vi "Data Save.vi"(11 "Data In":T2) -> (2 "Number":i32, 3 "Data Out":T2)   [LabVIEW 2020]
uses:
  Alin/QMH/000 Module Data Type.ctl
  Alin/QMH/Queue Message.ctl
  <vilib>/Utility/miscctls.llb/LVMapReplaceAction.ctl
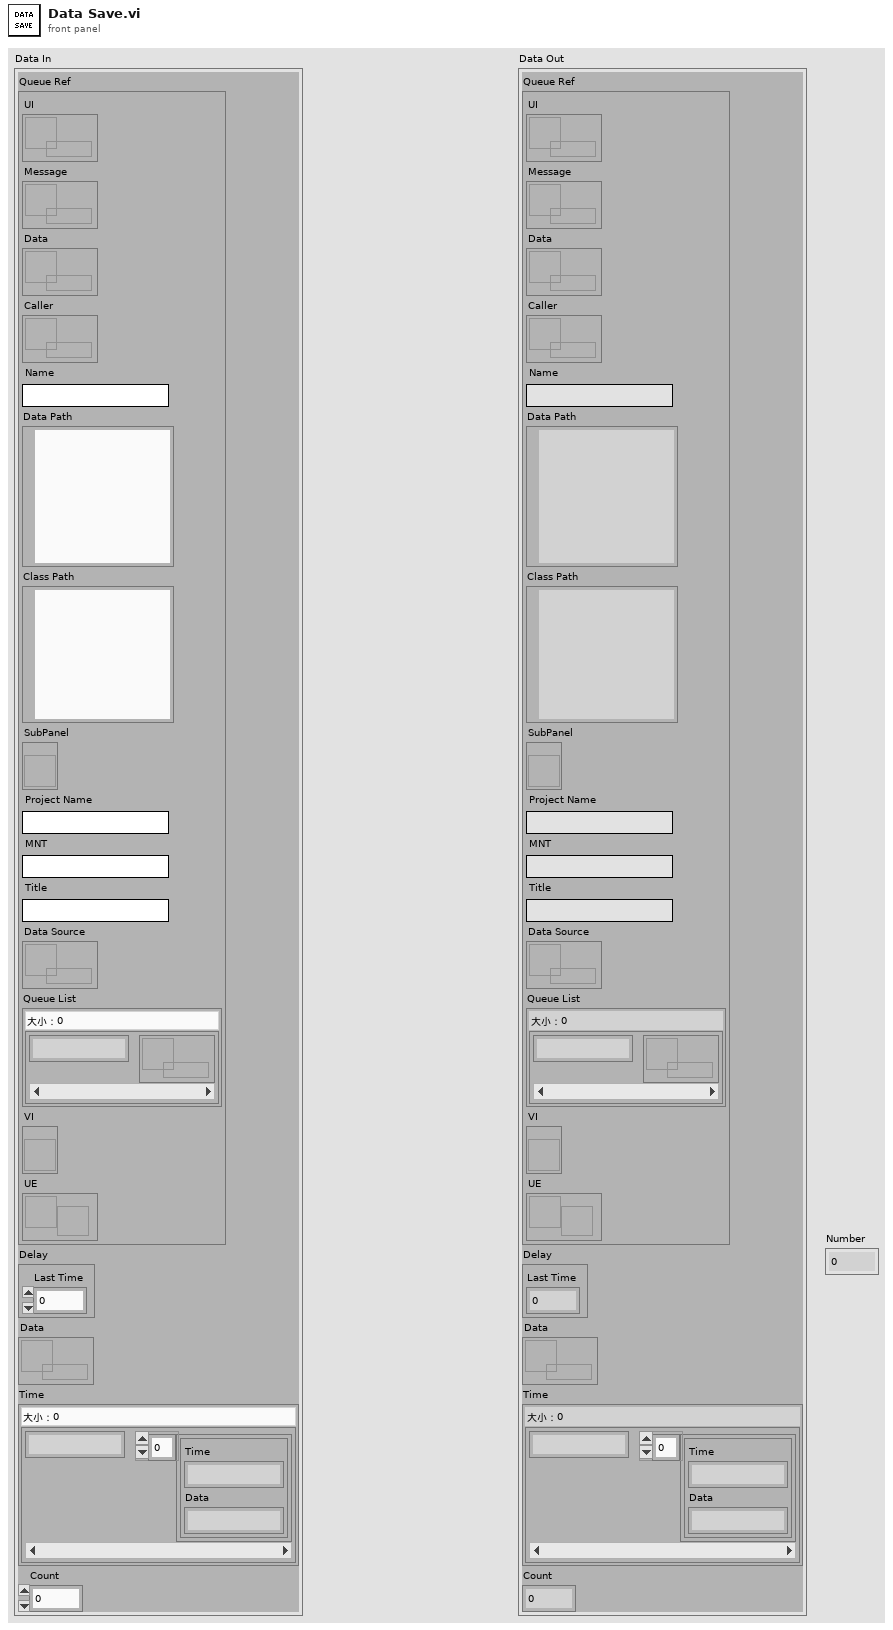
[diagram p1: front panel]
types:
  T1 = typedef "000 Module Data Type.ctl" = cluster{"UI":refnum<queue>, "Message":refnum<queue>, "Data":refnum<queue>, "Caller":refnum<queue>, "Name":string, "Data Path":path, "Class Path":path, "SubPanel":refnum<vi>, "Project Name":string, "MNT":string, "Title":string, "Data Source":refnum<queue>, "Queue List":map{string, refnum<queue>}, "VI":refnum<vi>, "UE":refnum<user-event>}
  T2 = cluster{"Queue Ref":T1, "Delay":cluster{"Last Time":dbl}, "Data":refnum<queue>, "Time":map{string, cluster{"Time":string, "Data":string}[]}, "Count":dbl}
  T3 = typedef "SDQ Data Type.ctl" = cluster{"CAN Length":string, "CAN Name":string, "CAN ID":string, "CAN Type":string, "Test Item":string, "Byte Order":string, "Instruction":string, "Control Type":string, "Group":string, "Offset":dbl, "Coefficient":dbl, "Write Enable":bool, "Lable Type":string, "Key?":string, "Set Value":string, "Upper":dbl, "Lower":dbl, "Unit":string, "Formula":string, "Test Item Type":string, "Length":i32, "Address":string, "Name":string, "Identifier":string, "Data Type":string, "Enumerate?":string, "Enumerate List":string, "Data":string, "Source":string}
  T4 = typedef "LVMapReplaceAction.ctl" = enum32{"Modify Entry only if found", "Add or Modify Entry", "Delete Entry"}
  T5 = map{string, cluster{"Time":string, "Data":string}[]}
  T6 = cluster{"Name":string, "Data":cluster{"Time":string, "Data":string}[]}
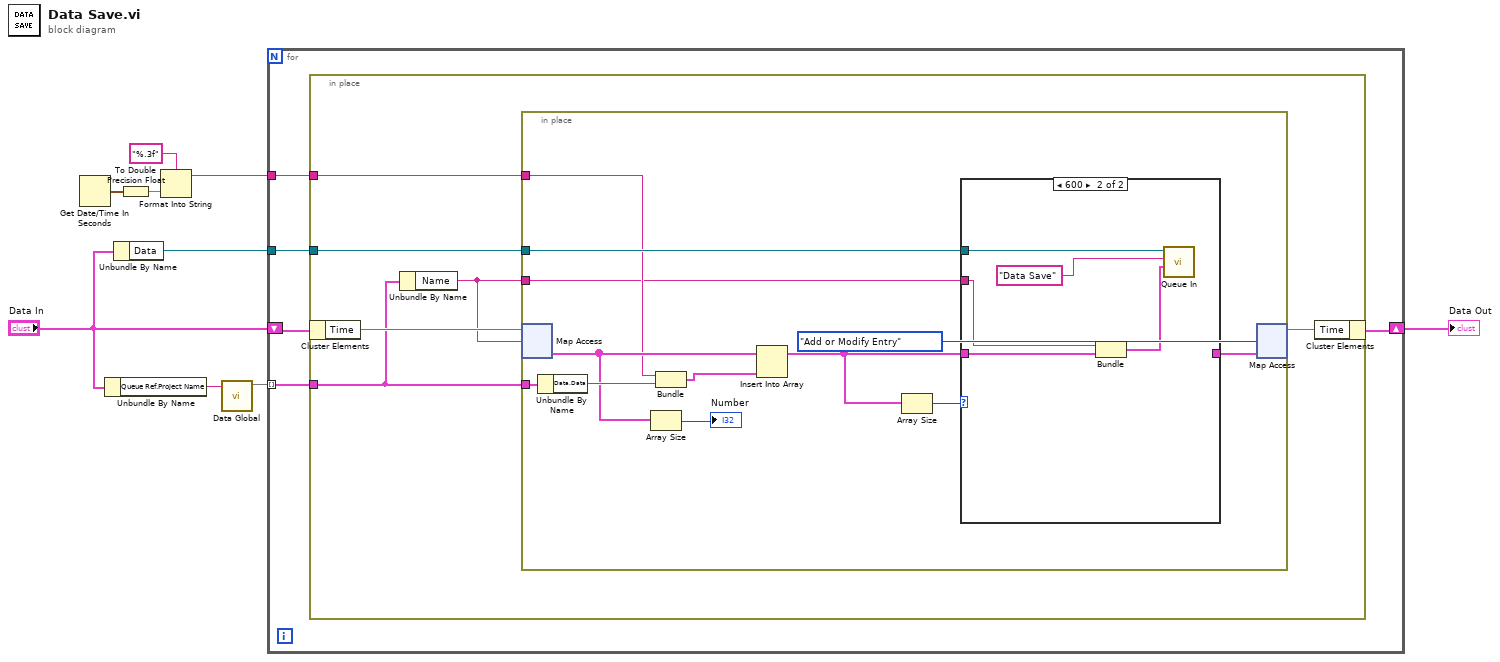
[diagram p0: block diagram]
diagram:
  n1 = Get Date/Time In Seconds() -> (seconds since 1Jan1904=w8:timestamp)
  n2 = Unbundle By Name("Data In") -> ("Queue Ref.Project Name"=w9:string)
  n3 = Unbundle By Name("Data In") -> ("Data"=w2:refnum<queue>)
  n4 = To Double Precision Float(number=w8) -> (double precision float=w6:dbl)
  n5 = Format Into String(format string="%.3f" ("格式字符串"), w6) -> (resulting string=w1:string)  [unwired: 2 in, 1 out]
  n6 = call "Data Global.vi"("Name"=w9) -> ("Data Out"=w7:map{string, T3})  [unwired: 7 in, 3 out]
  n7 = for {
    tunnel: w7 -> [w12] mode=indexing
    shift-right: [w14] -> w4
    shift-left: "Data In" -> [w13]
    tunnel: w2 -> [w11]
    tunnel: w1 -> [w10]
    n8 = in-place {
      in-place-border: w12 -> [w18]
      in-place-border: w11 -> [w17]
      in-place-border: w10 -> [w16]
      n9 = in-place-cluster #1(w13) -> ("Time"=w20:T5)
      n10 = Unbundle By Name(w18) -> ("Name"=w15:string)
      n11 = in-place {
        in-place-border: w18 -> [w32]
        in-place-border: w17 -> [w24]
        in-place-border: w16 -> [w23]
        in-place-border: w15 -> [w22]
        n12 = in-place-map #2(w20, w15) -> (w26:cluster{"Time":string, "Data":string}[])  [unwired: 1 in, 1 out]
        n13 = Unbundle By Name(w32) -> ("Data.Data"=w31:string)
        n14 = Array Size(array=w26) -> (size(s)=→"Number":i32)
        n15 = Bundle(w23, "Data"=w31) -> (w29:cluster{string, "Data":string})  [unwired: 1 in]
        n16 = Insert Into Array(array=w26, new element=w29) -> (w28:cluster{"Time":string, "Data":string}[])  [unwired: 1 in]
        n17 = Array Size(array=w28) -> (size(s)=w21:i32)
        n18 = case shown="600" w21 {
          tunnel: w28 -> [w33 w37]
          tunnel: [w33 _] -> w27
          tunnel: w24 -> [_ w35]
          tunnel: w22 -> [_ w34]
          frame 0, Default {
          }
          frame 600 {
            n19 = Bundle("Name"=w34, "Data"=w37) -> (w36:T6)  [unwired: 1 in]
            n20 = call "Queue In.vi"("Data"=w36, "Message"="Data Save", "Queue In"=w35) -> ()  [unwired: 7 in, 2 out]
          }
        }
        n21 = in-place-map #2(w27, LVMapReplaceAction."Add or Modify Entry" ("操作")) -> (w19:T5)  [unwired: 2 out]
      }
      n22 = in-place-cluster #1("Time"=w19) -> (w14:T2)
    }
  }
  "Data Out" <- w4
